vi "RSNRPZ Fetch Buffer Data.vi"(8 "error in (no error)":errorcluster, 9 "Array Size (0)":i32, 10 "Channel (1)":i32=1, 11 "VISA session":refnum<visa-resource-name> caption="VISA resource name") -> (0 "error out":errorcluster, 1 "Read Count":i32, 2 "Measurement Array":dbl[](array[numeric]) format="%.3p", 3 "dup VISA session":refnum<visa-resource-name> caption="VISA resource name")   [LabVIEW 2010]
doc: "This VI returns the buffer measurement the sensor acquires for the channel you specify. The measurement is from an acquisition that you previously initiated. \n\nYou use the RSNRPZ Initiate.vi to start an acquisition on the channels that you specify. You use the RSNRPZ Get Measurement Complete State.vi to determine when the acquisition is complete.\n\nYou can call the RSNRPZ Read Buffer Data.vi instead of the RSNRPZ Initiate.vi. The RSNRPZ Read Buffer Data.vi starts an acquisition, waits for the acquisition to complete, and returns the measurement for the channel you specify.\n\nNote:\n\n1) If the measurement is not available, acquistion has not been initialized or it's still in progress function retrune an error (0xBFFC0100 Measurement is not available)"
uses:
  rsnrpz_32.dll
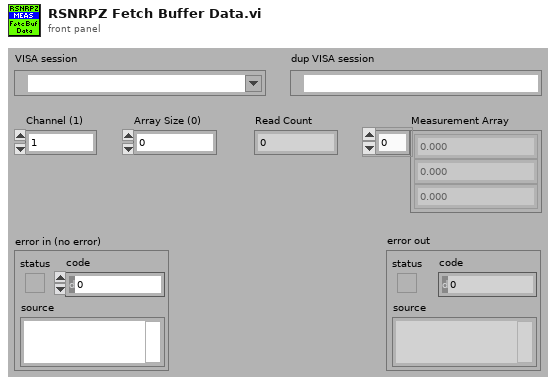
[diagram p1: front panel]
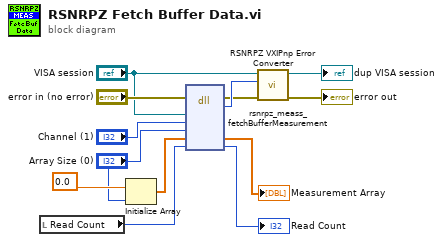
[diagram p0: block diagram]
diagram:
  n1 = local read "Read Count"() -> (w8:i32)
  n2 = Initialize Array(0.0, "Array Size (0)") -> (w10:dbl[])
  n3 = dll-call lib="rsnrpz_32.dll" fn="rsnrpz_meass_fetchBufferMeasurement"(error in="error in (no error)", "Instrument Handle"="VISA session", "Channel"="Channel (1)", "Array Size"="Array Size (0)", w10, "Read Count"=w8) -> (error out=w5:errorcluster, "Status"=w12:i32, →"Measurement Array":dbl[], "Read Count"=→"Read Count":i32)  [unwired: 5 in, 1 out]
  n4 = call <instrlib>:"RSNRPZ VXIPnp Error Converter.vi"("error in"=w5, "VXIPnp error code"=w12, "VISA session"="VISA session") -> ("error out"=→"error out":errorcluster, "dup VISA session"=→"dup VISA session":refnum<visa-resource-name>)  [unwired: 7 in]
